vi "Threshold and Centroid Image.vi"(0 "Raw Image":dbl[][](array[numeric]), 3 "Threshold or Threshold Fraction*":dbl=254.0) -> (4 "y":i32[](array[numeric]), 5 "sum":dbl, 6 "Thresholded Beam":dbl[][](array[numeric]), 7 "x0":dbl=2147483647.0, 8 "x":i32[](array[numeric]), 9 "y0":dbl=2147483647.0)   [LabVIEW 2020]
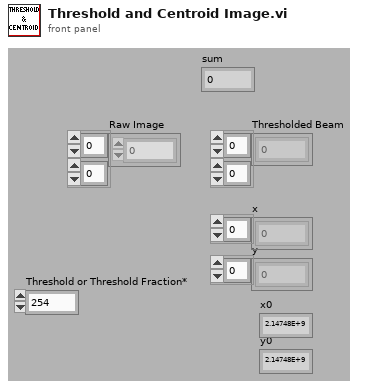
[diagram p1: front panel]
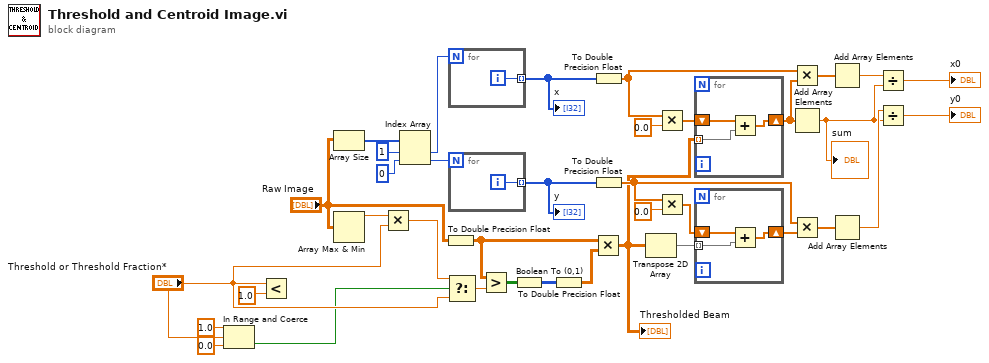
[diagram p0: block diagram]
diagram:
  n1 = In Range and Coerce(upper limit=1.0, x="Threshold or Threshold Fraction*", lower limit=0.0) -> (In Range?=w1:bool)  [unwired: 1 out]
  n2 = Less?(x="Threshold or Threshold Fraction*", y=1.0) -> ()  [unwired: 1 out]
  n3 = Array Size(array="Raw Image") -> (size(s)=w20:i32[])
  n4 = Array Max & Min(array="Raw Image") -> (max value=w10:dbl)  [unwired: 3 out]
  n5 = Multiply(x=w10, y="Threshold or Threshold Fraction*") -> (x*y=w8:dbl)
  n6 = Index Array(array=w20, index #1=1 ("index"), index #2=0 ("index")) -> (element #1=w21:i32, element #2=w22:i32)
  n7 = To Double Precision Float(number="Raw Image") -> (double precision float=w17:dbl[][])
  n8 = Select(t=w8, s=w1, f="Threshold or Threshold Fraction*") -> (s? t:f=w7:dbl)
  n9 = for {
    N: w21 -> [_]
    tunnel: [w38] -> w19 mode=indexing
    i -> [w38]
  }
  "x" <- w19
  n10 = for {
    N: w22 -> [_]
    tunnel: [w39] -> w18 mode=indexing
    i -> [w39]
  }
  "y" <- w18
  n11 = Greater?(x=w17, y=w7) -> (0:w23:bool[][])
  n12 = Boolean To (0,1)(Boolean=w23) -> (0, 1=w24:i16[][])
  n13 = To Double Precision Float(number=w24) -> (double precision float=w25:dbl[][])
  n14 = Multiply(x=w17, y=w25) -> (x*y=w14:dbl[][])
  "Thresholded Beam" <- w14
  n15 = To Double Precision Float(number=w19) -> (double precision float=w36:dbl[])
  n16 = To Double Precision Float(number=w18) -> (double precision float=w37:dbl[])
  n17 = Transpose 2D Array(2D array=w14) -> (transposed array=w13:dbl[][])
  n18 = Multiply(x=w36, y=0.0) -> (x*y=w29:dbl[])
  n19 = Multiply(x=w37, y=0.0) -> (x*y=w32:dbl[])
  n20 = for {
    tunnel: w14 -> [w41] mode=indexing
    shift-right: [w40] -> w30
    shift-left: w29 -> [w42]
    n21 = Add(x=w42, y=w41) -> (x+y=w40:dbl[])
  }
  n22 = for {
    tunnel: w13 -> [w44] mode=indexing
    shift-right: [w43] -> w31
    shift-left: w32 -> [w45]
    n23 = Add(x=w45, y=w44) -> (x+y=w43:dbl[])
  }
  n24 = Multiply(x=w36, y=w30) -> (x*y=w26:dbl[])
  n25 = Add Array Elements(numeric array=w30) -> (sum=w12:dbl)
  "sum" <- w12
  n26 = Multiply(x=w37, y=w31) -> (x*y=w35:dbl[])
  n27 = Add Array Elements(numeric array=w26) -> (sum=w27:dbl)
  n28 = Add Array Elements(numeric array=w35) -> (sum=w34:dbl)
  n29 = Divide(x=w27, y=w12) -> (x/y=→"x0":dbl)
  n30 = Divide(x=w34, y=w12) -> (x/y=→"y0":dbl)
